vi "PCP OFF With the Power.vi"(0 "PSU type":T1, 11 "error In":errorcluster) -> (15 "error out":errorcluster)   [LabVIEW 2011]
uses:
  PSU Type.ctl
  PCP Commands.ctl
  PCP Command definer.ctl
  Magna Interface/Magna Commands.ctl
  Magna Interface/Magna Command Definer.ctl
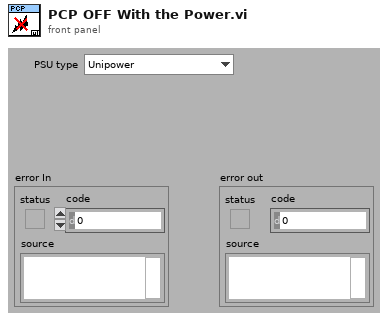
[diagram p1: front panel]
types:
  T1 = typedef "PSU Type.ctl" = enum16{"Unipower", "Magna 8.3A", "Magna 12A", "None"}
  T2 = typedef "PCP Commands.ctl" = enum16{"do not use HE - Help", "RDd - Most used inputs", "RA - All analog inputs", "RE n Reset DO n", "SE n Set DO n", "RP - Get digital inputs", "VA d Set AO A  Motor Volt", "VB d Set AO B  Cable Resistance", "VEr - Get Version", "DYp - Depth counter", "DR - Reset Depth Counter", "DS n Set Depth options(0-3)", "do not use ME - Manual mode enabled", "MD - Manual mode disabled", "ID - Get ID(2001)", "TS - Get Timestamp", "TO d(s)  Set timeout", "do not use LO n Start Loop Mode(1,2)", "AL n RD&LO variation", "ST - Stop Loop Mode"}
  T3 = typedef "PCP Command definer.ctl" = cluster{"Action":T2, "n(0)":i32, "d(0.0)":dbl}
  T4 = typedef "Magna Commands.ctl" = enum16{"Read Inputs", "HV ON", "HV OFF", "Set Resistance", "Set Head Voltage SP"}
  T5 = typedef "Magna Command Definer.ctl" = cluster{"Action":T4, "n(0)":i32, "d(0.0)":dbl}
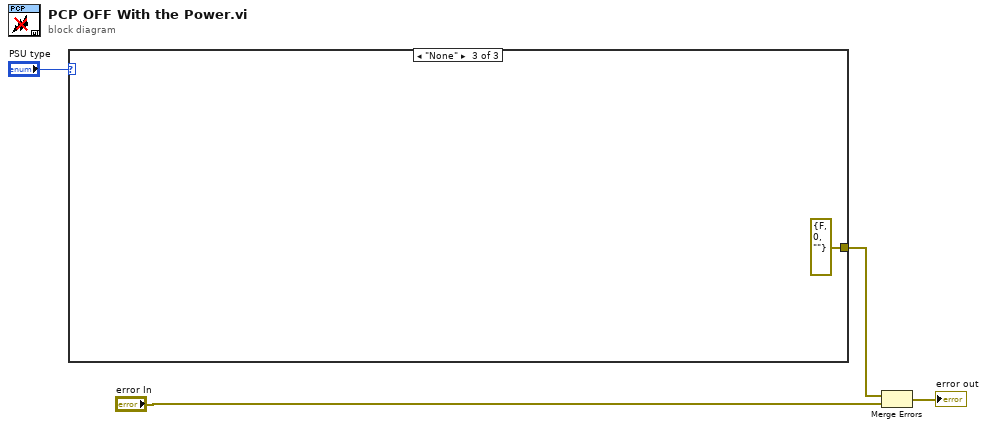
[diagram p0: block diagram]
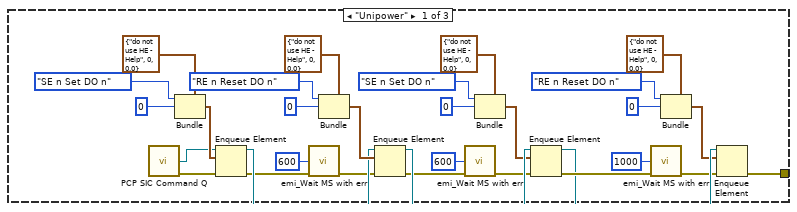
[diagram p2: hidden frame]
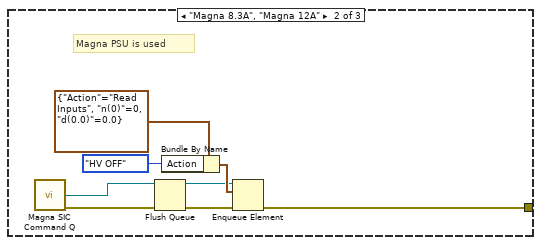
[diagram p3: hidden frame]
diagram:
  n1 = case shown="\"None\"" "PSU type" {
    tunnel: [w35 w40 errorcluster {"status"=FALSE, "code"=0, "source"=""} ("error out")] -> w4
    frame "Unipower" {
      n2 = call "PCP SIC Command Q.vi"() -> ("PCP cmd Q"=w6:refnum<queue>, "error out"=w5:errorcluster)  [unwired: 14 in]
      n3 = Bundle(cluster=T3 {"Action"=enum."do not use HE - Help", "n(0)"=0, "d(0.0)"=0.0} ("PCP command definer"), "Action"=PCP_Commands."SE n Set DO n", "n(0)"=0) -> (w12:T3)  [unwired: 1 in]
      n4 = Enqueue Element(queue=w6, element=w12, error in (no error)=w5) -> (queue out=w10:refnum<queue>, error out=w7:errorcluster)  [unwired: 1 in, 1 out]
      n5 = call "emi_Wait MS with err.vi"("milliseconds to wait(0)"=u32 600, "error in (no error)"=w7) -> ("error out"=w9:errorcluster)  [unwired: 13 in]
      n6 = Bundle(cluster=T3 {"Action"=enum."do not use HE - Help", "n(0)"=0, "d(0.0)"=0.0} ("PCP command definer"), "Action"=PCP_Commands."RE n Reset DO n", "n(0)"=0) -> (w14:T3)  [unwired: 1 in]
      n7 = Enqueue Element(queue=w10, element=w14, error in (no error)=w9) -> (queue out=w26:refnum<queue>, error out=w25:errorcluster)  [unwired: 1 in, 1 out]
      n8 = call "emi_Wait MS with err.vi"("milliseconds to wait(0)"=u32 600, "error in (no error)"=w25) -> ("error out"=w23:errorcluster)  [unwired: 13 in]
      n9 = Bundle(cluster=T3 {"Action"=enum."do not use HE - Help", "n(0)"=0, "d(0.0)"=0.0} ("PCP command definer"), "Action"=PCP_Commands."SE n Set DO n", "n(0)"=0) -> (w21:T3)  [unwired: 1 in]
      n10 = Enqueue Element(queue=w26, element=w21, error in (no error)=w23) -> (queue out=w33:refnum<queue>, error out=w34:errorcluster)  [unwired: 1 in, 1 out]
      n11 = call "emi_Wait MS with err.vi"("milliseconds to wait(0)"=u32 1000, "error in (no error)"=w34) -> ("error out"=w28:errorcluster)  [unwired: 13 in]
      n12 = Bundle(cluster=T3 {"Action"=enum."do not use HE - Help", "n(0)"=0, "d(0.0)"=0.0} ("PCP command definer"), "Action"=PCP_Commands."RE n Reset DO n", "n(0)"=0) -> (w30:T3)  [unwired: 1 in]
      n13 = Enqueue Element(queue=w33, element=w30, error in (no error)=w28) -> (error out=w35:errorcluster)  [unwired: 1 in, 2 out]
    }
    frame "Magna 8.3A", "Magna 12A" {
      # "Magna PSU is used"
      n14 = call "Magna SIC Command Q.vi"() -> ("queue out"=w37:refnum<queue>, "error out"=w39:errorcluster)  [unwired: 14 in]
      n15 = Flush Queue(queue=w37, error in (no error)=w39) -> (queue out=w36:refnum<queue>, error out=w38:errorcluster)  [unwired: 1 out]
      n16 = Bundle By Name(cluster=T5 {"Action"=enum."Read Inputs", "n(0)"=0, "d(0.0)"=0.0} ("element"), "Action"=Magna_Commands."HV OFF") -> (w42:T5)
      n17 = Enqueue Element(queue=w36, element=w42, error in (no error)=w38) -> (error out=w40:errorcluster)  [unwired: 1 in, 2 out]
    }
    frame "None" {
    }
  }
  n18 = Merge Errors(w4, "error In") -> (→"error out":errorcluster)
